vi "Write Target Field (T).vi"(8 "error in (no error)":errorcluster, 10 "Target Field (T)":dbl, 11 "Magnet in":refnum<class "Magnet.lvclass">) -> (0 "error out":errorcluster, 3 "Magnet out":refnum<class "Magnet.lvclass">)   [LabVIEW 2016, in "Magnet.lvclass"]
uses:
  Magnet.lvclass
  Magnet.lvclass/Magnet.ctl
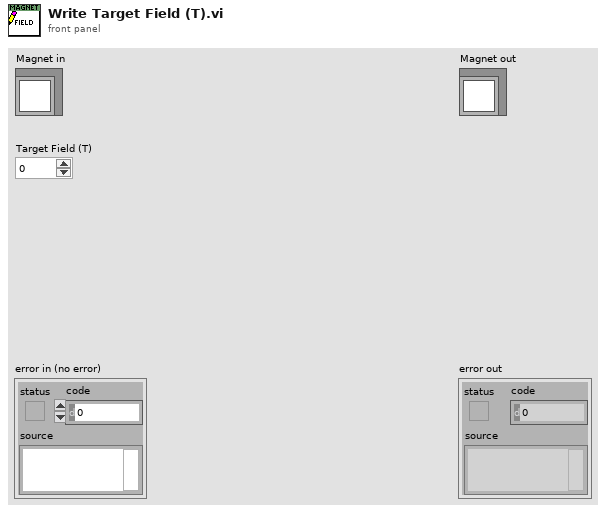
[diagram p1: front panel]
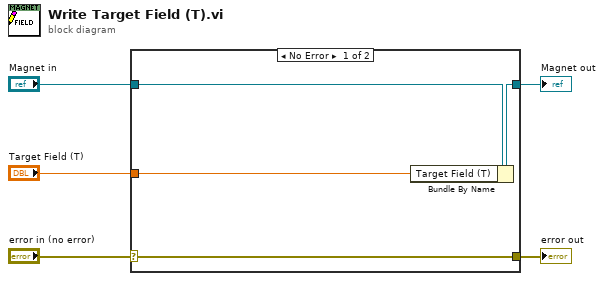
[diagram p0: block diagram]
diagram:
  n1 = case shown="No Error" "error in (no error)" {
    selector: "error in (no error)" -> [w9 w10]
    tunnel: [w9 w10] -> w4
    tunnel: [w7 w11] -> w2
    tunnel: "Magnet in" -> [w8 w11]
    tunnel: "Target Field (T)" -> [w6 _]
    frame No Error {
      n2 = Bundle By Name(cluster=w8, "Target Field (T)"=w6) -> (w7:refnum<class "Magnet.lvclass">)
    }
    frame Error {
    }
  }
  "error out" <- w4
  "Magnet out" <- w2
